vi "SendActionEvent.vi"(8 "error in (no error)":errorcluster, 9 "Variant":variant, 10 "Action":T1, 11 "WindowFrame in":refnum<class "WindowFrame.lvclass">) -> (0 "error out":errorcluster, 3 "WindowFrame out":refnum<class "WindowFrame.lvclass">)   [LabVIEW 2021, in "WindowFrame.lvlib" / "WindowFrame.lvclass"]
uses:
  WindowFrame.lvclass
  Action.ctl
  ActionData.ctl
  GetEventActionRef.vi
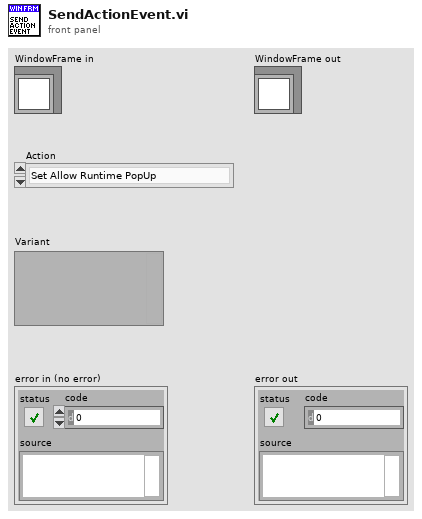
[diagram p1: front panel]
types:
  T1 = typedef "WindowFrame.lvlib/WindowFrame.lvclass/Action.ctl" = enum16{"Set Allow Runtime PopUp", "Set Behavior", "Set Closable", "Set Custom Title", "Set Highlight Return Button", "Set Is Frontmost", "Set Minimizable", "Set Minimum Size", "Set Monitor", "Set Resizable", "Set Panel Bounds", "Set Run VI Transparently", "Set Show Menu Bar", "Set State", "Set Title", "Set Title Bar Colors", "Set Title Bar Visible", "Set Transparancy", "Set Window Bounds", "Get Allow Runtime PopUp", "Get Behavior", "Get Closable", "Get Custom Title", "Get Highlight Return Button", "Get Is Frontmost", "Get Minimizable", "Get Minimum Size", "Get Monitor", "Get Panel Bounds", "Get Resizable", "Get Run VI Transparently", "Get Show Menu Bar", "Get State", "Get Title", "Get Title Bar Colors", "Get Title Bar Visible", "Get Transparancy", "Get Window Bounds", "--", "Center", "Close", "Open", "Run-Time Position:Centered", "Run-Time Position:Custom", "Run-Time Position:Get Position", "Run-Time Position:Maximized", "Run-Time Position:Minimized", "Run-Time Position:Unchanged", "---", "Insert VI", "Remove VI", "Insert VI Index", "Remove VI Index", "Exit"}
  T2 = typedef "WindowFrame.lvlib/WindowFrame.lvclass/ActionData.ctl" = cluster{"Action":T1, "Variant":variant}
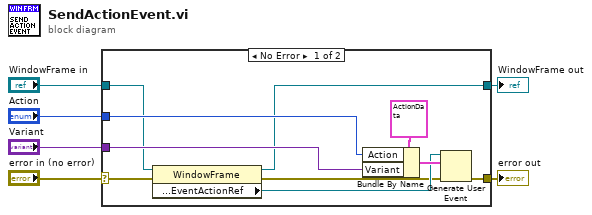
[diagram p0: block diagram]
diagram:
  n1 = case shown="No Error" "error in (no error)" {
    selector: "error in (no error)" -> [w9 w17]
    tunnel: "Action" -> [w16 _]
    tunnel: [w14 w17] -> w5
    tunnel: "WindowFrame in" -> [w11 w18]
    tunnel: [w7 w18] -> w3
    tunnel: "Variant" -> [w12 _]
    frame No Error {
      n2 = property class="WindowFrame"(reference=w11, error in=w9) -> (reference out=w7:refnum<class "WindowFrame.lvclass">, error out=w8:errorcluster, "Private:Properties:EventActionRef"=w10:refnum<user-event>)
      n3 = Bundle By Name(cluster=T2 {"Action"=enum."Set Allow Runtime PopUp", "Variant"=variant} ("event data"), "Action"=w16, "Variant"=w12) -> (w15:T2)
      n4 = Generate User Event(user event=w10, event data cluster=w15, error in=w8) -> (error out=w14:errorcluster)  [unwired: 1 in, 1 out]
    }
    frame Error {
    }
  }
  "error out" <- w5
  "WindowFrame out" <- w3
